vi "get path to CoreEngine dll.vi"() -> (8 "path to wavekit library":path, 12 "Release/Debug":string)   [LabVIEW 2020]
uses:
  <vilib>/registry/registry.llb/Registry RtKey.ctl
  <vilib>/registry/registry.llb/Registry SAM.ctl
  <vilib>/registry/registry.llb/Read Registry Value Simple STR.vi
panel:
  in  "error in (no error)":errorcluster
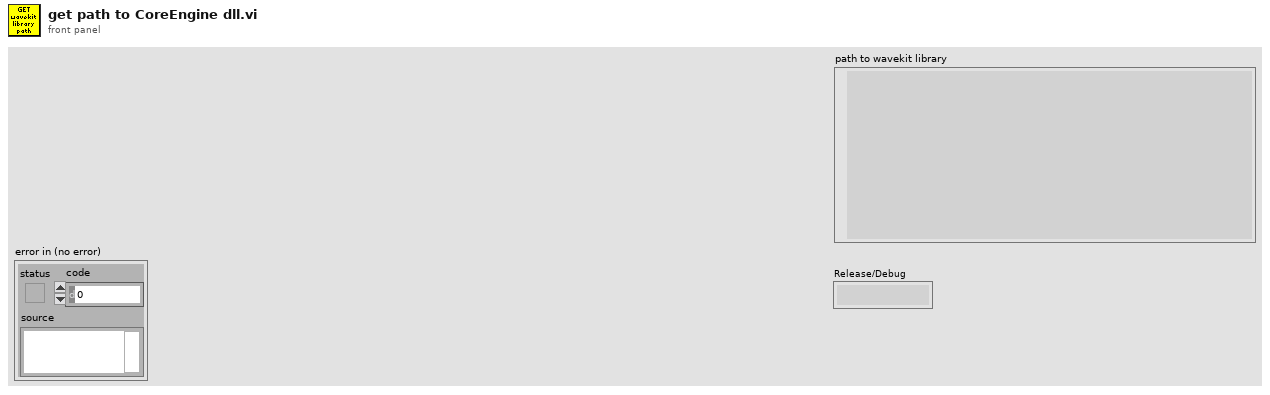
[diagram p1: front panel]
types:
  T1 = typedef "Registry SAM.ctl" = enum32{"KEY_QUERY_VALUE", "KEY_SET_VALUE", "KEY_CREATE_SUB_KEY", "KEY_ENUMERATE_SUB_KEYS", "KEY_NOTIFY", "KEY_CREATE_LINK", "KEY_READ", "KEY_WRITE", "KEY_ALL_ACCESS", "KEY_READ | KEY_WRITE"}
  T2 = typedef "Registry RtKey.ctl" = enum32{"HKEY_CLASSES_ROOT", "HKEY_CURRENT_USER", "HKEY_LOCAL_MACHINE", "HKEY_USERS", "HKEY_PERFORMANCE_DATA", "HKEY_CURRENT_CONFIG", "HKEY_DYN_DATA"}
  T3 = enum32{"invalid app kind", "Development System", "Run Time System", "Student Edition", "Embedded LabVIEW", "Evaluation", "Custom"}
  T4 = typedef "Registry refnum.ctl" = refnum<k1>
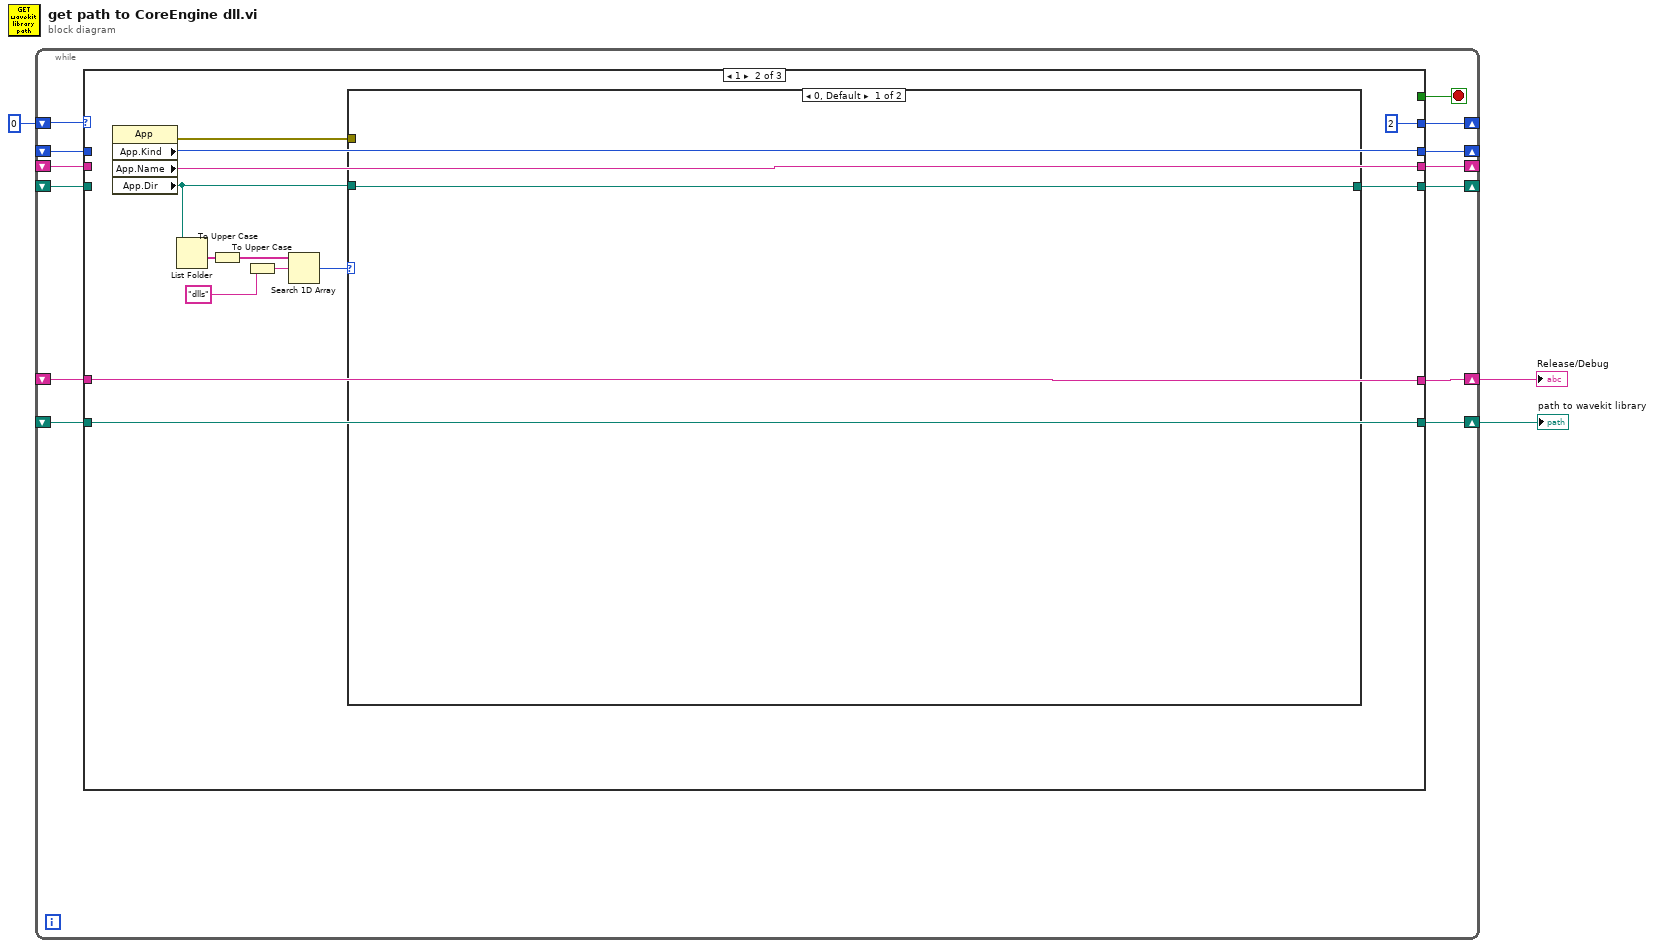
[diagram p0: block diagram]
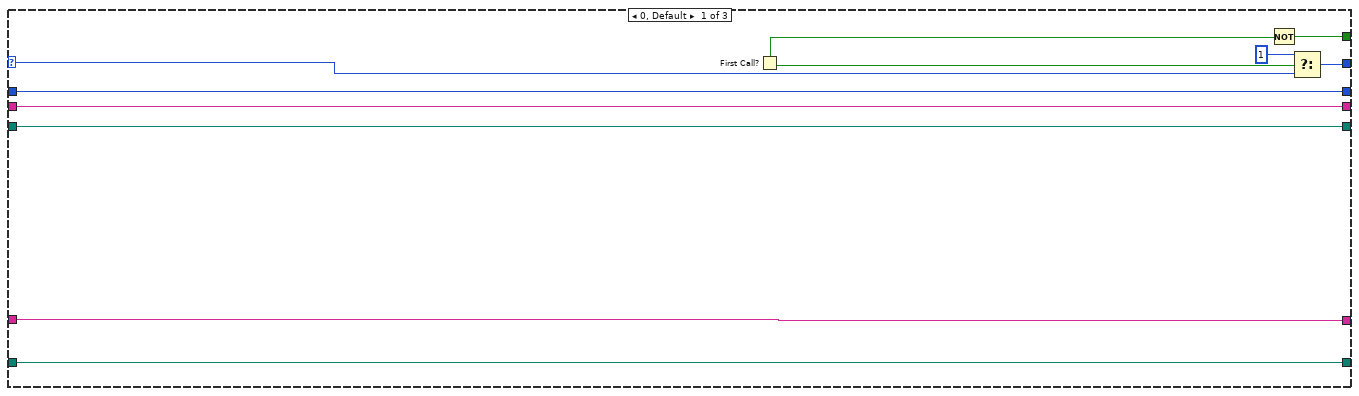
[diagram p2: hidden frame]
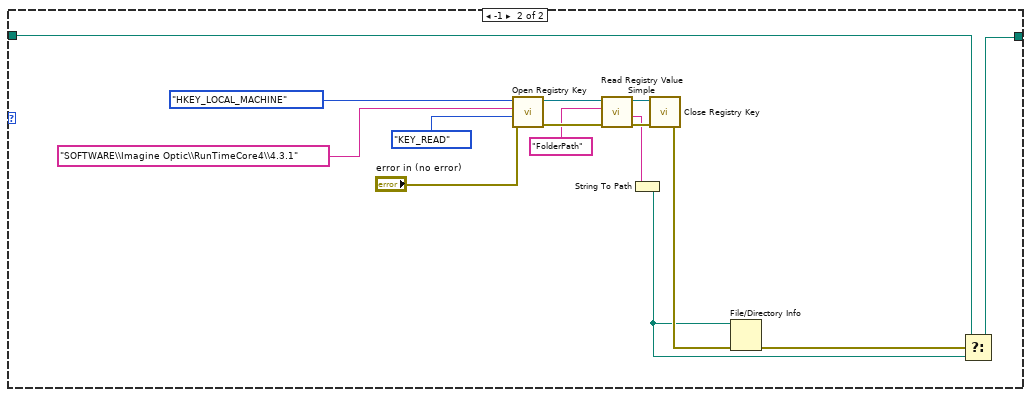
[diagram p3: hidden frame]
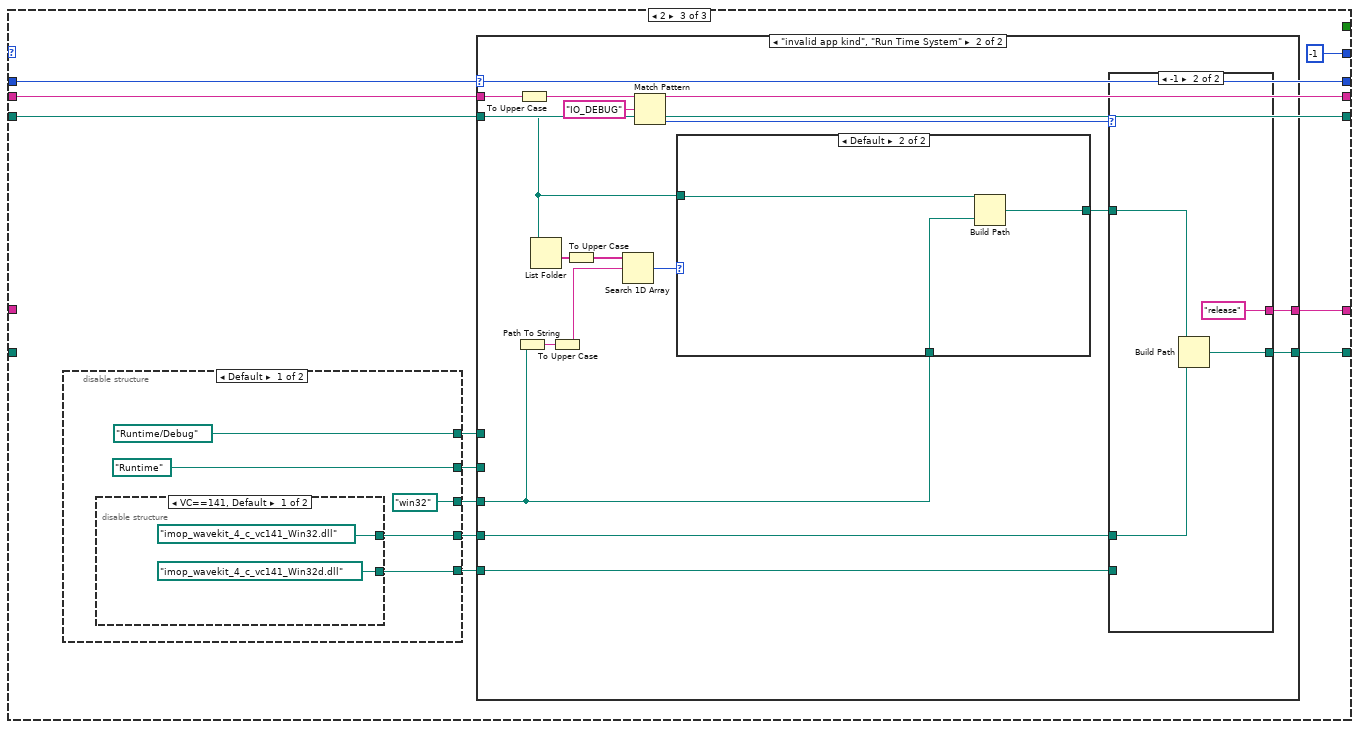
[diagram p4: hidden frame]
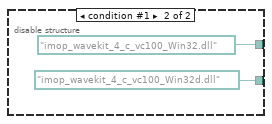
[diagram p5: hidden frame]
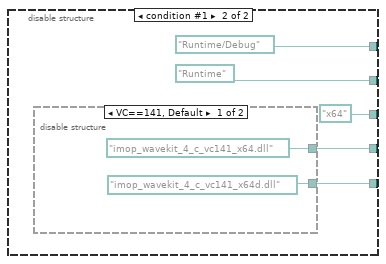
[diagram p6: hidden frame]
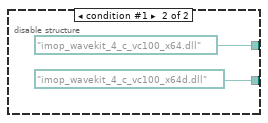
[diagram p7: hidden frame]
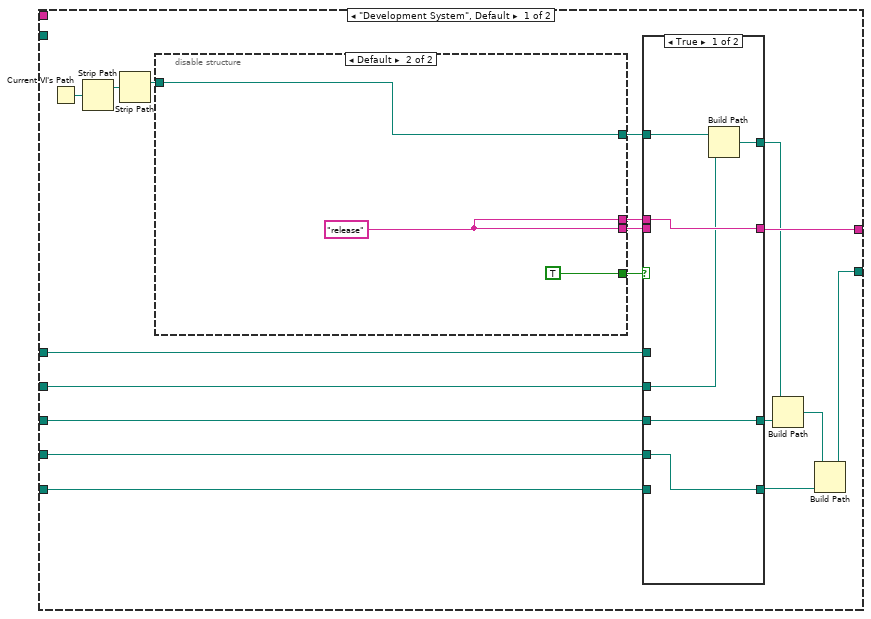
[diagram p8: hidden frame]
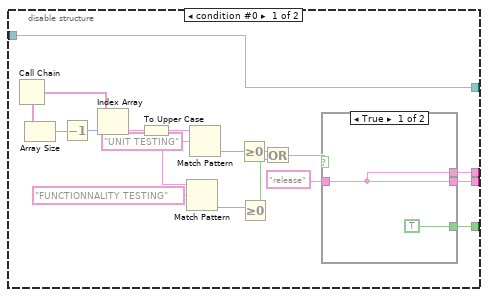
[diagram p9: hidden frame]
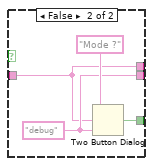
[diagram p10: hidden frame]
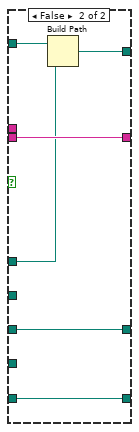
[diagram p11: hidden frame]
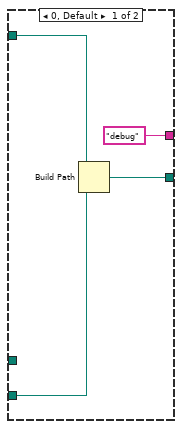
[diagram p12: hidden frame]
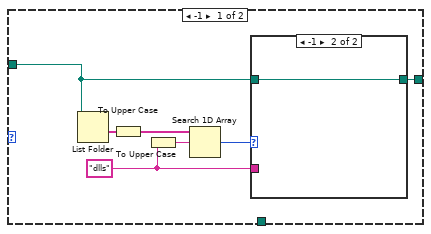
[diagram p13: hidden frame]
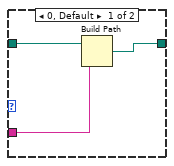
[diagram p14: hidden frame]
diagram:
  n1 = while {
    shift-right: [w14] -> _
    shift-left: 0 -> [w15]
    shift-right: [w12] -> _
    shift-left: _ -> [w9]
    shift-right: [w11] -> _
    shift-left: _ -> [w10]
    shift-right: [w16] -> w3
    shift-left: _ -> [w8]
    shift-right: [w7] -> w1
    shift-left: _ -> [w6]
    shift-right: [w5] -> _
    shift-left: _ -> [w4]
    stop <- w13 stop-if-true
    n2 = case shown="1" w15 {
      selector: w15 -> [w23 _ _]
      tunnel: [w19 w36 w66] -> w16
      tunnel: [w26 2 -1] -> w14
      tunnel: [w22 _ _] -> w13
      tunnel: [w21 w38 w64] -> w12
      tunnel: [w20 w37 w63] -> w11
      tunnel: w10 -> [w20 _ w63]
      tunnel: w9 -> [w21 _ w64]
      tunnel: w8 -> [w19 w36 _]
      tunnel: [w18 w35 w62] -> w7
      tunnel: w6 -> [w18 w35 _]
      tunnel: [w17 w34 w56] -> w5
      tunnel: w4 -> [w17 _ w56]
      frame 0, Default {
        n3 = First Call?() -> (First Call?: T/F=w24:bool)
        n4 = Not(x=w24) -> (.not. x?=w22:bool)
        n5 = Select(t=1, s=w24, f=w23) -> (s? t:f=w26:i32)
      }
      frame 1 {
        n6 = property class="App"() -> (error out=w27:errorcluster, "App.Kind"=w38:T3, "App.Name"=w34:string, "App.Dir"=w29:path)  [unwired: 2 in, 1 out]
        n7 = List Folder(path=w29) -> (folder names=w33:string[])  [unwired: 3 in, 3 out]
        n8 = To Upper Case(1:w33) -> (0:w32:string[])
        n9 = To Upper Case(1:"dlls" ("element")) -> (0:w30:string)
        n10 = Search 1D Array(1D array=w32, element=w30) -> (index of element=w28:i32)  [unwired: 1 in]
        n11 = case shown="0, Default" w28 {
          tunnel: [w40 w46] -> w37
          tunnel: w29 -> [w40 w43]
          tunnel: w27 -> [_ _]
          frame 0, Default {
          }
          frame -1 {
            n12 = call <vilib>:"Open Registry Key.vi"("error in (no error)"="error in (no error)", "security access mask (KEY_READ | KEY_WRITE)"=Registry_SAM."KEY_READ", "subkey"="SOFTWARE\\Imagine Optic\\RunTimeCore4\\4.3.1", "root key (HKEY_LOCAL_MACHINE)"=Registry_RtKey."HKEY_LOCAL_MACHINE") -> ("error out"=w53:errorcluster, "refnum out"=w52:T4)  [unwired: 6 in]
            n13 = call-poly <vilib>:"Read Registry Value Simple.vi"("error in (no error)"=w53, "value"="FolderPath", "refnum"=w52) -> ("error out"=w48:errorcluster, "String/Binary data"=w47:string, "refnum out"=w51:T4)  [unwired: 3 in, 1 out]
            n14 = String To Path(string=w47) -> (path=w42:path)
            n15 = call <vilib>:"Close Registry Key.vi"("error in (no error)"=w48, "refnum"=w51) -> ("error out"=w45:errorcluster)  [unwired: 5 in]
            n16 = File/Directory Info(path=w42, error in=w45) -> (error out=w41:errorcluster)  [unwired: 6 out]
            n17 = Select(t=w43, s=w41, f=w42) -> (s? t:f=w46:path)
          }
        }
      }
      frame 2 {
        n18 = disable-structure shown="Default" {
          disable-tunnel: [w69 w80] -> w58
          disable-tunnel: [path "Runtime" ("path in") path "Runtime" ("path in")] -> w60
          disable-tunnel: [path "Runtime/Debug" ("path in") path "Runtime/Debug" ("path in")] -> w61
          disable-tunnel: [w68 w77] -> w57
          disable-tunnel: [path "win32" ("path in") path "x64" ("path in")] -> w59
          frame condition #0 (active) {
            n19 = disable-structure shown="VC==141, Default" {
              disable-tunnel: [path "imop_wavekit_4_c_vc141_Win32.dll" ("path in") path "imop_wavekit_4_c_vc100_Win32.dll" ("path in")] -> w69
              disable-tunnel: [path "imop_wavekit_4_c_vc141_Win32d.dll" ("path in") path "imop_wavekit_4_c_vc100_Win32d.dll" ("path in")] -> w68
              frame condition #0 (active) {
              }
              frame condition #1 {
              }
            }
          }
          frame condition #1 {
            n20 = disable-structure shown="VC==141, Default" {
              disable-tunnel: [path "imop_wavekit_4_c_vc141_x64.dll" ("path in") path "imop_wavekit_4_c_vc100_x64.dll" ("path in")] -> w80
              disable-tunnel: [path "imop_wavekit_4_c_vc141_x64d.dll" ("path in") path "imop_wavekit_4_c_vc100_x64d.dll" ("path in")] -> w77
              frame condition #0 (active) {
              }
              frame condition #1 {
              }
            }
          }
        }
        n21 = case shown="\"invalid app kind\", \"Run Time System\"" w64 {
          tunnel: [w101 w156] -> w62
          tunnel: w63 -> [_ w155]
          tunnel: [w102 w154] -> w66
          tunnel: w58 -> [w100 w147]
          tunnel: w60 -> [w99 _]
          tunnel: w61 -> [w98 _]
          tunnel: w57 -> [w97 w143]
          tunnel: w59 -> [w86 w141]
          tunnel: w56 -> [_ w146]
          frame "Development System", Default {
            n22 = Current VI's Path() -> (path=w92:path)
            n23 = Strip Path(path=w92) -> (stripped path=w93:path)  [unwired: 1 out]
            n24 = Strip Path(path=w93) -> (stripped path=w90:path)  [unwired: 1 out]
            n25 = disable-structure shown="Default" {
              disable-tunnel: [w119 TRUE ("T button?")] -> w96
              disable-tunnel: [w118 w127] -> w95
              disable-tunnel: [w117 w127] -> w94
              disable-tunnel: [w103 w126] -> w91
              disable-tunnel: w90 -> [w103 w126]
              frame condition #0 {
                n26 = Call Chain() -> (call chain=w116:string[])
                n27 = Array Size(array=w116) -> (size(s)=w115:i32)
                n28 = Decrement(x=w115) -> (x-1=w114:i32)
                n29 = Index Array(array=w116, index=w114) -> (element=w113:string)
                n30 = To Upper Case(1:w113) -> (0:w110:string)
                n31 = Match Pattern(string=w110, regular expression="FUNCTIONNALITY TESTING") -> (offset past match=w107:i32)  [unwired: 1 in, 3 out]
                n32 = Match Pattern(string=w110, regular expression="UNIT TESTING") -> (offset past match=w108:i32)  [unwired: 1 in, 3 out]
                n33 = Greater Or Equal To 0?(x=w108) -> (x >= 0?=w106:bool)
                n34 = Greater Or Equal To 0?(x=w107) -> (x >= 0?=w105:bool)
                n35 = Or(x=w106, y=w105) -> (x .or. y?=w104:bool)
                n36 = case shown="True" w104 {
                  tunnel: [TRUE ("T button?") w125] -> w119
                  tunnel: [w121 w122] -> w118
                  tunnel: [w121 w123] -> w117
                  tunnel: "release" ("T button name (\"OK\")") -> [w121 w122]
                  frame True {
                  }
                  frame False {
                    w123 = "debug" ("F button name (\"Cancel\")")
                    n37 = Two Button Dialog(message="Mode ?", 1:w123, 2:w122) -> (T button?=w125:bool)
                  }
                }
              }
              frame condition #1 (active) {
                w127 = "release" ("T button name (\"OK\")")
              }
            }
            n38 = case shown="True" w96 {
              tunnel: [w134 w140] -> w102
              tunnel: w95 -> [w134 _]
              tunnel: w94 -> [_ w140]
              tunnel: w91 -> [w133 w139]
              tunnel: [w132 w138] -> w88
              tunnel: w99 -> [w131 _]
              tunnel: w98 -> [_ w137]
              tunnel: w100 -> [w130 _]
              tunnel: [w130 w136] -> w89
              tunnel: w97 -> [_ w136]
              tunnel: w86 -> [w129 w135]
              tunnel: [w129 w135] -> w85
              frame True {
                n39 = Build Path(base path=w133, name or relative path=w131) -> (appended path=w132:path)
              }
              frame False {
                n40 = Build Path(base path=w139, name or relative path=w137) -> (appended path=w138:path)
              }
            }
            n41 = Build Path(base path=w88, name or relative path=w85) -> (appended path=w87:path)
            n42 = Build Path(base path=w87, name or relative path=w89) -> (appended path=w101:path)
          }
          frame "invalid app kind", "Run Time System" {
            n43 = Path To String(path=w141) -> (string=w149:string)
            n44 = To Upper Case(1:w146) -> (0:w142:string)
            n45 = List Folder(path=w155) -> (folder names=w153:string[])  [unwired: 3 in, 3 out]
            n46 = To Upper Case(1:w149) -> (0:w148:string)
            n47 = To Upper Case(1:w153) -> (0:w152:string[])
            n48 = Search 1D Array(1D array=w152, element=w148) -> (index of element=w151:i32)  [unwired: 1 in]
            n49 = Match Pattern(string=w142, regular expression="IO_DEBUG") -> (offset past match=w144:i32)  [unwired: 1 in, 3 out]
            n50 = case shown="Default" w151 {
              tunnel: [w168 w177] -> w150
              tunnel: w155 -> [w169 w176]
              tunnel: w141 -> [_ w178]
              frame -1 {
                w166 = "dlls" ("element")
                n51 = List Folder(path=w169) -> (folder names=w171:string[])  [unwired: 3 in, 3 out]
                n52 = To Upper Case(1:w171) -> (0:w167:string[])
                n53 = To Upper Case(1:w166) -> (0:w165:string)
                n54 = Search 1D Array(1D array=w167, element=w165) -> (index of element=w170:i32)  [unwired: 1 in]
                n55 = case shown="-1" w170 {
                  tunnel: [w172 w175] -> w168
                  tunnel: w169 -> [w174 w175]
                  tunnel: w166 -> [w173 _]
                  frame 0, Default {
                    n56 = Build Path(base path=w174, name or relative path=w173) -> (appended path=w172:path)
                  }
                  frame -1 {
                  }
                }
              }
              frame Default {
                n57 = Build Path(base path=w176, name or relative path=w178) -> (appended path=w177:path)
              }
            }
            n58 = case shown="-1" w144 {
              tunnel: [w160 w164] -> w156
              tunnel: ["debug" ("T button name (\"OK\")") "release" ("T button name (\"OK\")")] -> w154
              tunnel: w150 -> [w158 w162]
              tunnel: w147 -> [_ w161]
              tunnel: w143 -> [w157 _]
              frame 0, Default {
                n59 = Build Path(base path=w158, name or relative path=w157) -> (appended path=w160:path)
              }
              frame -1 {
                n60 = Build Path(base path=w162, name or relative path=w161) -> (appended path=w164:path)
              }
            }
          }
        }
      }
    }
  }
  "path to wavekit library" <- w1
  "Release/Debug" <- w3
